vi "Lock cells.vi"(0 "Display State In":T1, 5 "Cell":cluster{"Row":i32, "Column":i32}[](array[cluster]), 7 "Locked?":bool, 9 "Container State":T6, 11 "error in (no error)":errorcluster) -> (4 "Display State Out":T1, 15 "error out":errorcluster)   [LabVIEW 2015, in "KTable.xctl"]
uses:
  KTable.xctl
  <vilib>/_xctls/Container State.ctl
  State.ctl
  ColumnSpec.ctl
  ColumnType.ctl
  Table Properties.ctl
  Events.ctl
  Event Data.ctl
  Event Type.ctl
  <vilib>/_xctls/XControlSupport.lvlib
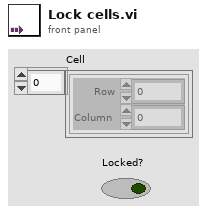
[diagram p1: front panel]
types:
  T1 = typedef "KTable.xctl/State.ctl" = cluster{"Columns":T2[], "Listbox":refnum<vi>, "Default row":string[], "Properties":T4, "Events":T5, "Locked":bool[][], "Size":cluster{"Rows":i32, "Columns":i32}, "rings":i32[][], "DefColors":u32[]}
  T2 = typedef "KTable.xctl/ColumnSpec.ctl" = cluster{"Name":string, "Type":T3, "Width":i32, "Strings":string[], "Position":enum16{"Left", "Center", "Right"}, "locked":bool, "cds":cluster{"Strings":string[]}[][]}
  T3 = typedef "KTable.xctl/ColumnType.ctl" = enum16{"String", "Enum", "Int", "Double", "Boolean", "Ring", "Formula", "Color"}
  T4 = typedef "KTable.xctl/Table Properties.ctl" = cluster{"Vertical scrollbar":bool, "User add/delete":bool, "Max rows":i32, "Row headers":bool}
  T5 = typedef "KTable.xctl/Events.ctl" = cluster{"Items Changed":refnum<user-event>}
  T6 = typedef "XControlSupport.lvlib/Container State.ctl" = cluster{"Indicator?":bool, "Run Mode?":bool, " Refnum":refnum<vi>}
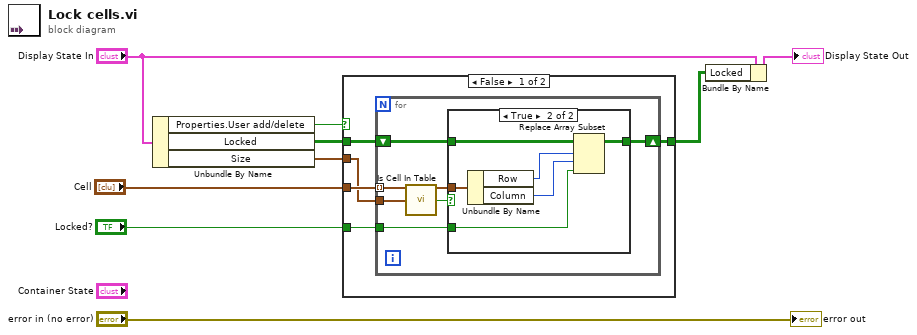
[diagram p0: block diagram]
diagram:
  n1 = Unbundle By Name("Display State In") -> ("Properties.User add/delete"=w7:bool, "Locked"=w6:bool[][], "Size"=w1:cluster{"Rows":i32, "Columns":i32})
  n2 = case shown="False" w7 {
    tunnel: w6 -> [w13 w29]
    tunnel: "Cell" -> [w14 _]
    tunnel: "Locked?" -> [w12 _]
    tunnel: [w11 w29] -> w2
    tunnel: w1 -> [w10 _]
    frame False {
      n3 = for {
        tunnel: w14 -> [w18] mode=indexing
        shift-right: [w20] -> w11
        shift-left: w13 -> [w21]
        tunnel: w12 -> [w19]
        tunnel: w10 -> [w16]
        n4 = call "Is Cell In Table.vi"("Cell"=w18, "Size"=w16) -> ("Cell thru"=w17:cluster{"Row":i32, "Column":i32}, "in table"=w15:bool)  [unwired: 12 in]
        n5 = case shown="True" w15 {
          tunnel: w21 -> [w22 w28]
          tunnel: [w22 w27] -> w20
          tunnel: w19 -> [_ w24]
          tunnel: w17 -> [_ w23]
          frame False {
          }
          frame True {
            n6 = Unbundle By Name(w23) -> ("Row"=w26:i32, "Column"=w25:i32)
            n7 = Replace Array Subset(array=w28, new element=w24, index (row)=w26, index (col)=w25) -> (w27:bool[][])
          }
        }
      }
    }
    frame True {
    }
  }
  n8 = Bundle By Name(cluster="Display State In", "Locked"=w2) -> (→"Display State Out":T1)
  "error out" <- "error in (no error)"
